vi "TEST Read Sweep nums this file.vi"(11 "ExistingFilePath":path=path "C:/Users/Public/Documents/UCAR/APAR Board Test/DataFiles/2015-07-31_17_36_0455.csv") -> (0 "error out":errorcluster, 1 "Num Sweeps":i32, 2 "Timestamp in s vs index in current file":i32[](graph), 3 "Sweep Number vs index in current file":i32[](graph), 5 "spreadsheet string":string)   [LabVIEW 2019, in "FileMerge.lvclass"]
uses:
  FileMerge.lvclass
  ExistingFileMgr/ExistingFileMgr.lvclass
  Sequence/SequenceSubvis/RF Direction.ctl
  Sequence/SequenceSubvis/PolarizationSelect.ctl
  Datalog/DatalogSubvis/SearchableTag.ctl
  Datalog/DataLog.lvclass
panel:
  in  "stop":bool
  out "i":i32
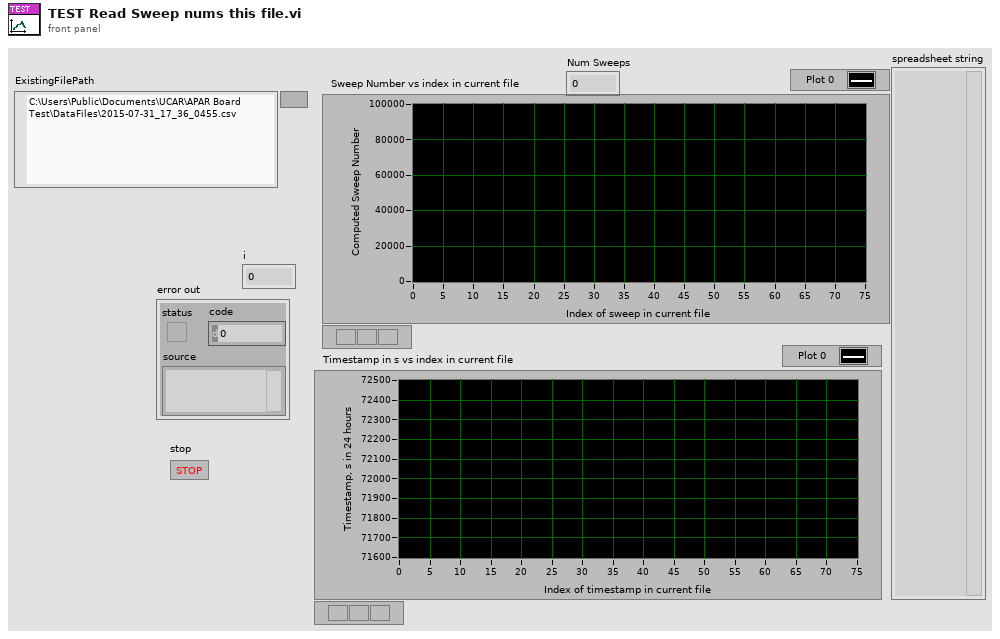
[diagram p1: front panel]
types:
  T1 = typedef "DataLog.lvclass/SearchableTag.ctl" = cluster{"Module, 0-63":i32, "RF Direction Tx0":T2, "Polarization, V0 H1":T3, "PhaseShift, deg":dbl, "Atten, dB":dbl}
  T2 = typedef "RF Direction.ctl" = enum16{"Tx - RF In", "Rx - RF Out"}
  T3 = typedef "PolarizationSelect.ctl" = enum16{"Vertical", "Horizontal"}
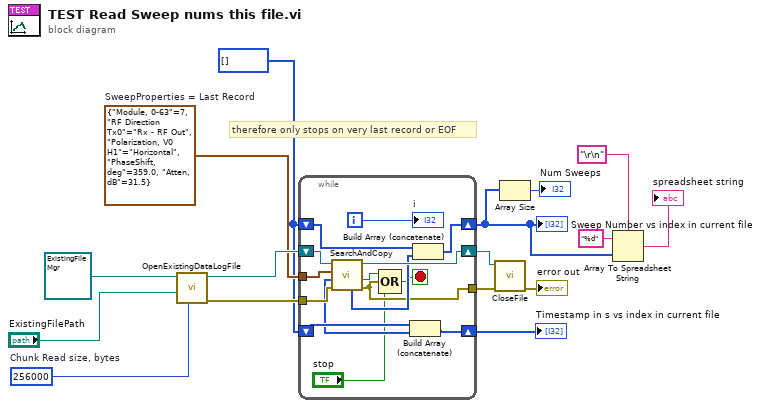
[diagram p0: block diagram]
diagram:
  w7 = 256000  # Chunk Read size, bytes
  w13 = T1 {"Module, 0-63"=7, "RF Direction Tx0"=enum."Rx - RF Out", "Polarization, V0 H1"=enum."Horizontal", "PhaseShift, deg"=359.0, "Atten, dB"=31.5}  # SweepProperties = Last Record
  w6 = i32[] []
  # "therefore only stops on very last record or EOF"
  n1 = call "OpenExistingDataLogFile.vi"("Chunk Read size, bytes"=w7, "ExistingFilePath"="ExistingFilePath", "ExistingFileMgr in"=refnum<class "ExistingFileMgr.lvclass"> refnum ("ExistingFileMgr.lvclass")) -> ("error out"=w12:errorcluster, "ExistingFileMgr out"=w14:refnum<class "ExistingFileMgr.lvclass">)  [unwired: 7 in]
  n2 = while {
    tunnel: w13 -> [w29]
    shift-right: [w30] -> w10
    shift-left: w14 -> [w31]
    shift-right: [w22] -> w4
    shift-left: w6 -> [w27]
    tunnel: w12 -> [w25]
    tunnel: [w18] -> w11
    shift-right: [w21] -> w5
    shift-left: w6 -> [w20]
    i -> [w26]
    stop <- w23 stop-if-true
    n3 = call "SearchAndCopy.vi"("error in (no error)"=w25, "SectionProperties"=w29, "ExistingFileMgr in"=w31) -> ("error out"=w18:errorcluster, "Found index or EOF"=w24:bool, "ExistingFileMgr out"=w30:refnum<class "ExistingFileMgr.lvclass">, "Sweep Nums"=w28:i32[], "Timestamps"=w19:i32[])  [unwired: 4 out]
    n4 = Compound Arithmetic op=OR(w24, w18, "stop") -> (w23:bool)
    n5 = Build Array (concatenate)(w20, w19) -> (w21:i32[])
    n6 = Build Array (concatenate)(w27, w28) -> (w22:i32[])
    "i" <- w26
  }
  "Sweep Number vs index in current file" <- w4
  "Timestamp in s vs index in current file" <- w5
  n7 = call "CloseFile.vi"("error in (no error)"=w11, "ExistingFileMgr in"=w10) -> ("error out"=→"error out":errorcluster)  [unwired: 8 in, 1 out]
  n8 = Array Size(array=w4) -> (size(s)=→"Num Sweeps":i32)
  n9 = Array To Spreadsheet String(delimiter (Tab)="\r\n", array=w4, 3:"%d" ("format string")) -> (spreadsheet string=→"spreadsheet string":string)
